vi "Fast Scan Get Data Curve.vi"(3 "Start Index":i32, 4 "Curve Number":i32, 5 "Conncection ID in":T1) -> (0 "Size of Double Array":i32, 1 "Double Array":dbl[](array[numeric]), 2 "Conncection ID out":T1)   [LabVIEW 2013]
uses:
  DeCoF SubVI Library/subVIs/DeCoF connection.ctl
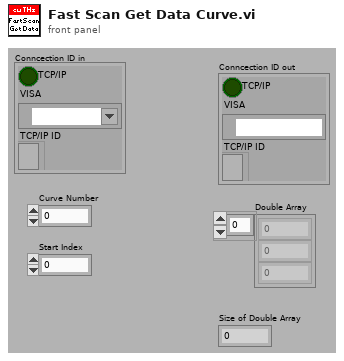
[diagram p1: front panel]
types:
  T1 = typedef "DeCoF connection.ctl" = cluster{"TCP/IP":bool, "VISA":refnum<visa-resource-name>, "TCP/IP ID":refnum<k5>}
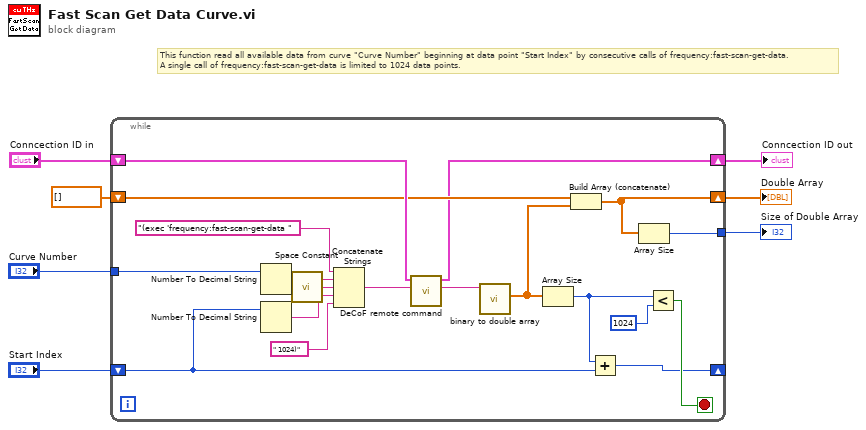
[diagram p0: block diagram]
diagram:
  # "This function read all available data from curve \"Curve Number\" beginning at data point \"Start Index\" by consecutive calls of frequency:fast-scan-get-data.\nA single call of frequency:fast-scan-get-data is limited to 1024 data points."
  n1 = while {
    tunnel: "Curve Number" -> [w23]
    shift-right: [w9] -> w4
    shift-left: dbl[] [] ("Double Array") -> [w15]
    shift-right: [w12] -> _
    shift-left: "Start Index" -> [w13]
    shift-right: [w10] -> w2
    shift-left: "Conncection ID in" -> [w25]
    tunnel: [w8] -> w1
    stop <- w16 stop-if-true
    n2 = Number To Decimal String(number=w23) -> (decimal integer string=w22:string)  [unwired: 1 in]
    n3 = Number To Decimal String(number=w13) -> (decimal integer string=w20:string)  [unwired: 1 in]
    n4 = call <vilib>:"Space Constant.vi"() -> ("String"=w21:string)
    n5 = Concatenate Strings("(exec 'frequency:fast-scan-get-data " ("param-name"), w22, w21, w20, " 1024)" ("param-name")) -> (w18:string)
    n6 = call "DeCoF remote command.vi"("command"=w18, "Conncection ID in"=w25) -> ("answer string"=w26:string, "Conncection ID out"=w10:T1)  [unwired: 3 in, 3 out]
    n7 = call "binary to double array.vi"("Binary String"=w26) -> ("Double Array"=w14:dbl[])  [unwired: 8 in, 2 out]
    n8 = Array Size(array=w14) -> (size(s)=w11:i32)
    n9 = Build Array (concatenate)(w15, w14) -> (w9:dbl[])
    n10 = Add(x=w11, y=w13) -> (x+y=w12:i32)
    n11 = Array Size(array=w9) -> (size(s)=w8:i32)
    n12 = Less?(x=w11, y=1024) -> (x < y?=w16:bool)
  }
  "Double Array" <- w4
  "Conncection ID out" <- w2
  "Size of Double Array" <- w1
